vi "Facade.vi"(0 "Data In":T4, 2 "Display State In":T2={"Color 1"=0, "Color 2"=0, "Direction"=enum."Top to Bottom", "Frame Color"=16777216, "Fraction"=0.0}, 3 "Container State":T3) -> (6 "Data Out":T4, 7 "Display State Out":T2={"Color 1"=0, "Color 2"=0, "Direction"=enum."Top to Bottom", "Frame Color"=16777216, "Fraction"=0.0}, 8 "Action":T1)   [LabVIEW 2020, in "KBackground Gradient.xctl"]
uses:
  KBackground Gradient.xctl
  Data.vi
  <vilib>/_xctls/Container State.ctl
  State.vi
  <vilib>/_xctls/Action.ctl
  <vilib>/_xctls/XControlSupport.lvlib
panel:
  out "Intensity Graph 2":i32[][](graph)
  out "Intensity Graph":i32[][](graph)
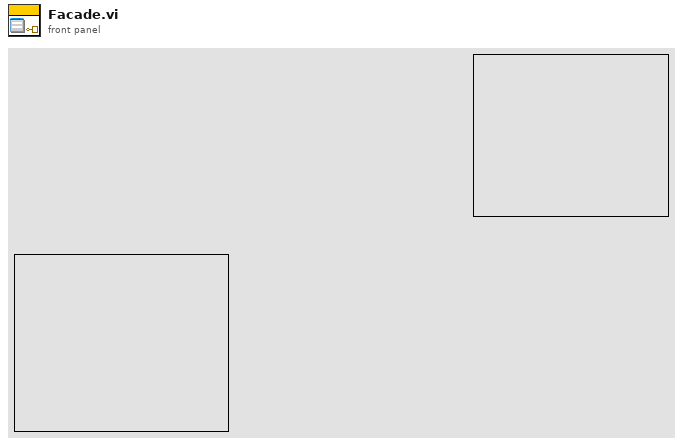
[diagram p1: front panel]
types:
  T1 = typedef "XControlSupport.lvlib/Action.ctl" = cluster{"Data Changed?":bool, "State Changed?":bool, "Action Name":string}
  T2 = typedef "KBackground Gradient.xctl/State.vi" = cluster{"Color 1":u32, "Color 2":u32, "Direction":enum16{"Top to Bottom", "Bottom to Top", "Left to Right", "Right to Left"}, "Frame Color":u32, "Fraction":dbl}
  T3 = typedef "XControlSupport.lvlib/Container State.ctl" = cluster{"Indicator?":bool, "Run Mode?":bool, " Refnum":refnum<vi>}
  T4 = typedef "KBackground Gradient.xctl/Data.vi" = dbl
  T5 = enum16{"Top to Bottom", "Bottom to Top", "Left to Right", "Right to Left"}
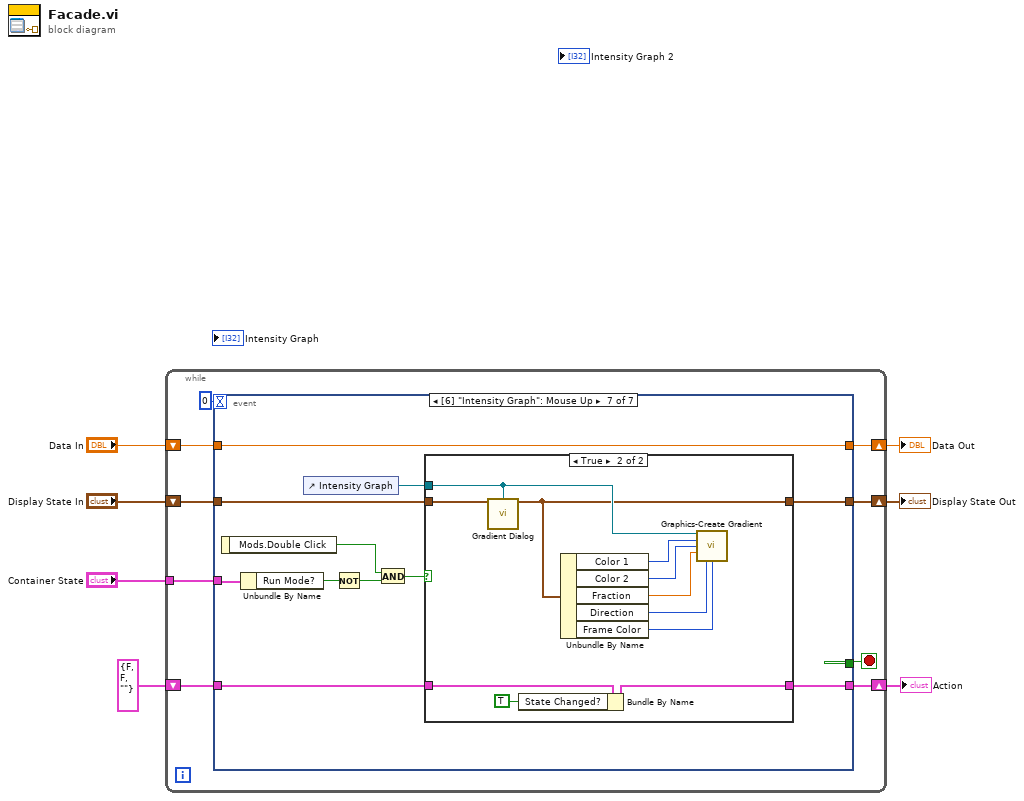
[diagram p0: block diagram]
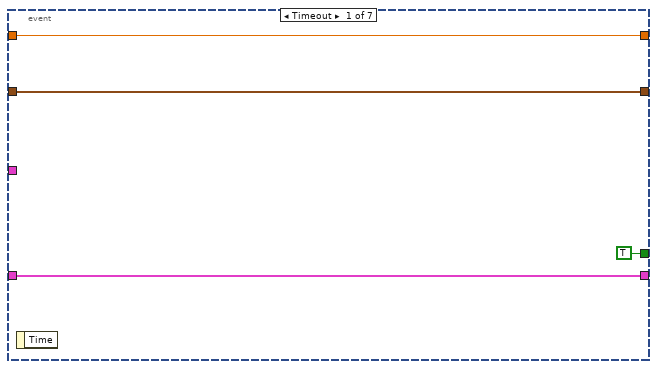
[diagram p2: hidden frame]
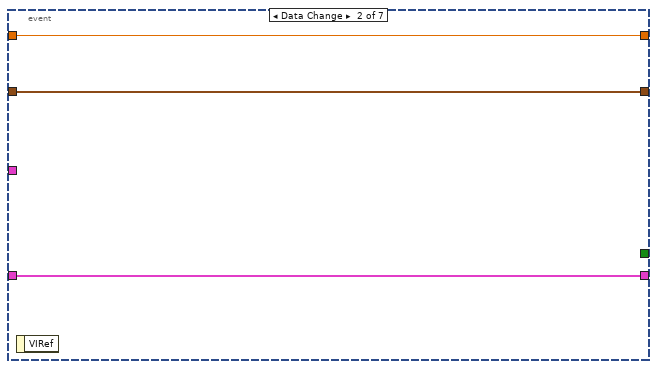
[diagram p3: hidden frame]
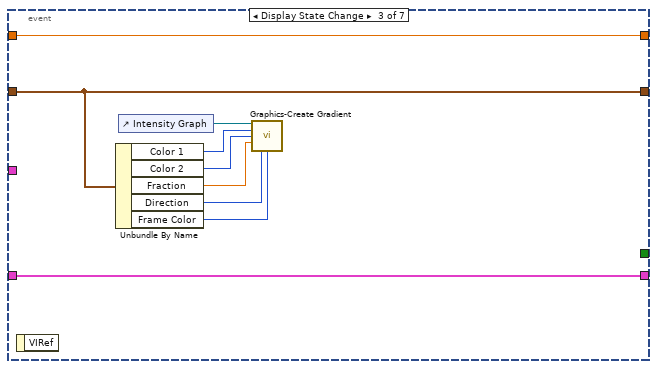
[diagram p4: hidden frame]
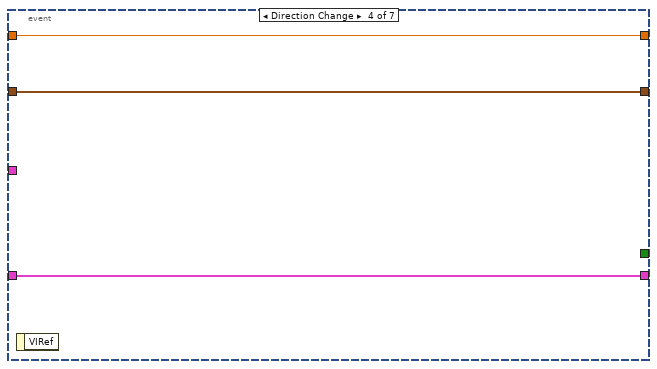
[diagram p5: hidden frame]
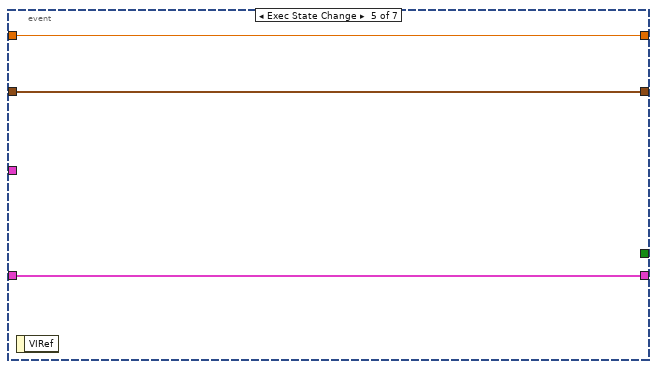
[diagram p6: hidden frame]
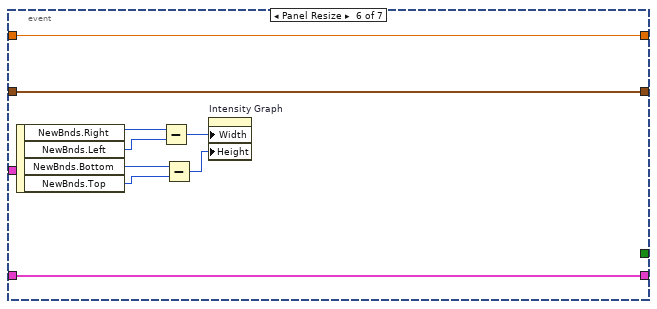
[diagram p7: hidden frame]
diagram:
  n1 = while {
    shift-right: [w15] -> w4
    shift-left: "Display State In" -> [w16]
    tunnel: "Container State" -> [w12]
    shift-right: [w10] -> w7
    shift-left: "Data In" -> [w11]
    shift-right: [w8] -> w2
    shift-left: T1 {"Data Changed?"=FALSE, "State Changed?"=FALSE, "Action Name"=""} ("Action") -> [w9]
    stop <- w14 stop-if-true
    n2 = event shown="[6] \"Intensity Graph\": Mouse Up" {
      selector: _ -> [_ _ _ _ _ _ _]
      dyn-events: _ -> [_ _ _ _ _ _ _]
      timeout: 0 -> [_ _ _ _ _ _ _]
      tunnel: w16 -> [w18 w22 w30 w35 w38 w47 w51]
      tunnel: [w18 w22 w30 w35 w38 w47 w48] -> w15
      tunnel: [TRUE _ _ _ _ _ _] -> w14
      tunnel: w12 -> [_ _ _ _ _ _ w57]
      tunnel: w11 -> [w17 w23 w32 w34 w37 w46 w58]
      tunnel: [w17 w23 w32 w34 w37 w46 w58] -> w10
      tunnel: [w19 w21 w31 w33 w36 w45 w49] -> w8
      tunnel: w9 -> [w19 w21 w31 w33 w36 w45 w50]
      event Timeout {
        n3 = event-data() -> ()  [unwired: 1 in, 1 out]
      }
      event Data Change {
        n4 = event-data() -> ()  [unwired: 1 in, 1 out]
      }
      event Display State Change {
        n5 = event-data() -> ()  [unwired: 1 in, 1 out]
        n6 = Unbundle By Name(w30) -> ("Color 1"=w28:u32, "Color 2"=w27:u32, "Fraction"=w26:dbl, "Direction"=w25:T5, "Frame Color"=w24:u32)
        n7 = control-ref of="Intensity Graph"() -> (w29:refnum<vi>)
        n8 = call "Graphics-Create Gradient.vi"("intensity graph"=w29, "Color 1"=w28, "Color 2"=w27, "Fraction"=w26, "Direction"=w25, "Frame Color"=w24) -> ()  [unwired: 9 in, 1 out]
      }
      event Direction Change {
        n9 = event-data() -> ()  [unwired: 1 in, 1 out]
      }
      event Exec State Change {
        n10 = event-data() -> ()  [unwired: 1 in, 1 out]
      }
      event Panel Resize {
        n11 = event-data() -> ("NewBnds.Right"=w42:i16, "NewBnds.Left"=w41:i16, "NewBnds.Bottom"=w40:i16, "NewBnds.Top"=w39:i16)  [unwired: 1 in]
        n12 = Subtract(x=w42, y=w41) -> (x-y=w43:i16)
        n13 = Subtract(x=w40, y=w39) -> (x-y=w44:i16)
        n14 = property on="Intensity Graph" class="IntGraph (strict)"("Width"=w43, "Height"=w44) -> ()  [unwired: 2 in, 2 out]
      }
      event "Intensity Graph": Mouse Up {
        n15 = event-data() -> ("Mods.Double Click"=w54:bool)  [unwired: 1 in]
        n16 = Unbundle By Name(w57) -> ("Run Mode?"=w56:bool)
        n17 = control-ref of="Intensity Graph"() -> (w52:refnum<vi>)
        n18 = Not(x=w56) -> (.not. x?=w55:bool)
        n19 = And(x=w54, y=w55) -> (x .and. y?=w53:bool)
        n20 = case shown="True" w53 {
          tunnel: w52 -> [_ w62]
          tunnel: w51 -> [w59 w71]
          tunnel: w50 -> [w60 w70]
          tunnel: [w60 w69] -> w49
          tunnel: [w59 w61] -> w48
          frame False {
          }
          frame True {
            n21 = call "Gradient Dialog.vi"("State In"=w71, "Control"=w62) -> ("State Out"=w61:T2)  [unwired: 13 in]
            n22 = Bundle By Name(cluster=w70, "State Changed?"=TRUE) -> (w69:T1)
            n23 = Unbundle By Name(w61) -> ("Color 1"=w63:u32, "Color 2"=w64:u32, "Fraction"=w65:dbl, "Direction"=w66:T5, "Frame Color"=w67:u32)
            n24 = call "Graphics-Create Gradient.vi"("intensity graph"=w62, "Color 1"=w63, "Color 2"=w64, "Fraction"=w65, "Direction"=w66, "Frame Color"=w67) -> ()  [unwired: 9 in, 1 out]
          }
        }
      }
    }
  }
  "Display State Out" <- w4
  "Data Out" <- w7
  "Action" <- w2
